vi "Handle Progress Bar.vi"(8 "error in":errorcluster, 10 "Numeric":i32, 11 ".NET Refnum in":refnum<k24>) -> (0 "error out":errorcluster, 3 ".NET Refnum out":refnum<k24>)   [LabVIEW 2014, in "Initialization and IO Node Scripting.lvlib"]
uses:
  Initialization and IO Node Scripting.lvlib
  System.Windows.Forms
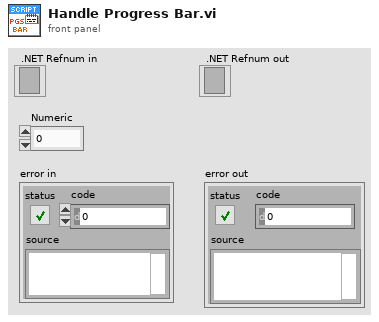
[diagram p1: front panel]
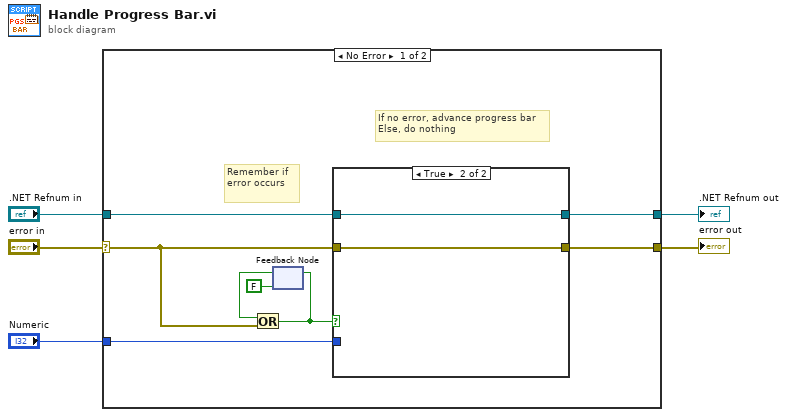
[diagram p0: block diagram]
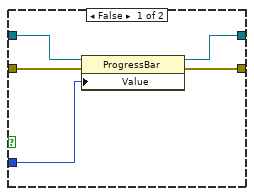
[diagram p2: hidden frame]
diagram:
  n1 = case shown="No Error" "error in" {
    selector: "error in" -> [w7 w21]
    tunnel: ".NET Refnum in" -> [w13 w22]
    tunnel: "Numeric" -> [w12 _]
    tunnel: [w11 w22] -> w3
    tunnel: [w6 w21] -> w1
    frame No Error {
      # "If no error, advance progress bar\nElse, do nothing"
      # "Remember if error occurs"
      n2 = feedback #1(FALSE) -> (w8:bool)
      n3 = Or(x=w8, y=w7) -> (x .or. y?=w10:bool)
      n4 = feedback-in #1(w10) -> ()
      n5 = case shown="True" w10 {
        tunnel: w12 -> [w16 _]
        tunnel: [w18 w20] -> w11
        tunnel: w13 -> [w17 w20]
        tunnel: w7 -> [w15 w19]
        tunnel: [w14 w19] -> w6
        frame False {
          n6 = property class="ProgressBar"(reference=w17, error in=w15, "Value"=w16) -> (reference out=w18:refnum<k24>, error out=w14:errorcluster)
        }
        frame True {
        }
      }
    }
    frame Error {
    }
  }
  ".NET Refnum out" <- w3
  "error out" <- w1
